vi "Input_channels.vi"(10 "Range":dbl=10.0) -> (0 "error out":errorcluster, 3 "Refnum out":refnum<k21>)   [LabVIEW 2021]
uses:
  <vilib>/DAQmx/create/scale.llb/DAQmx Create Scale (Linear).vi
  <vilib>/DAQmx/create/channels.llb/DAQmx Create Channel (AI-Voltage-Basic).vi
panel:
  out "Numeric":i32
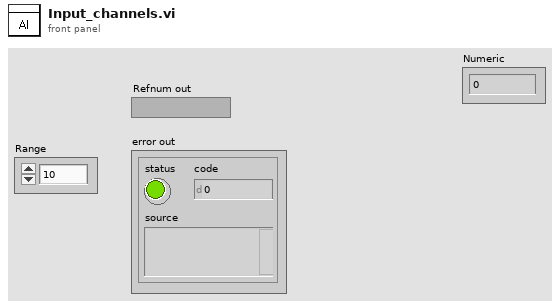
[diagram p1: front panel]
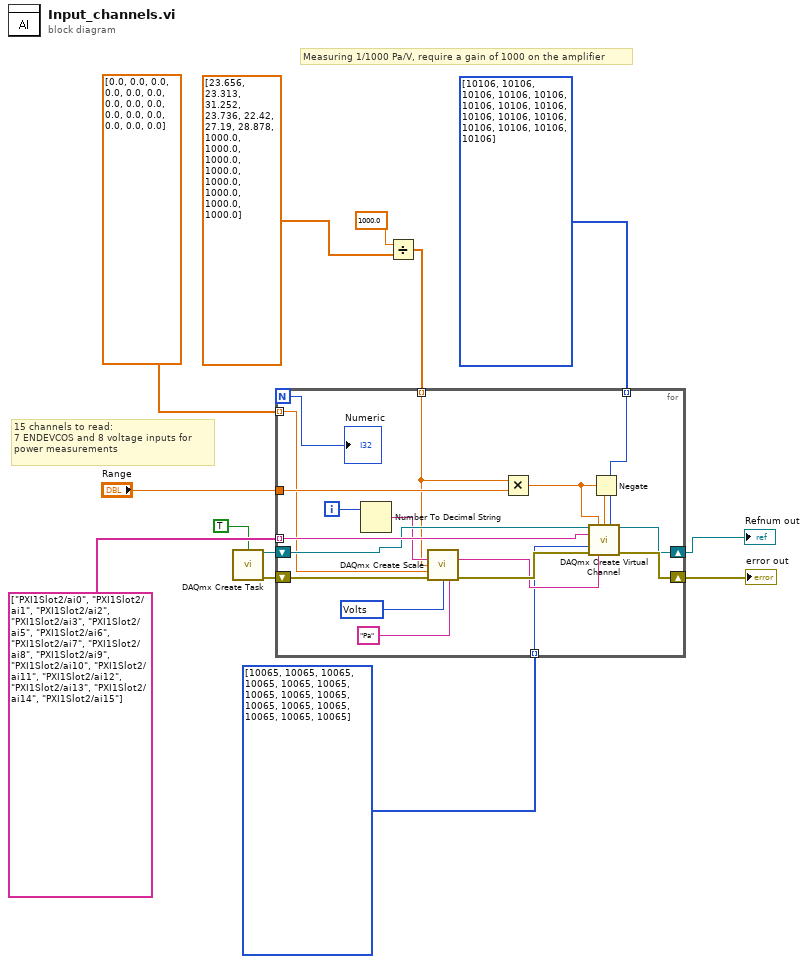
[diagram p0: block diagram]
diagram:
  w5 = i32[] [10065, 10065, 10065, 10065, 10065, 10065, 10065, 10065, 10065, 10065, 10065, 10065, 10065, 10065, 10065] items=["Volts"=10348, "From TEDS"=12516, "From Custom Scale"=10065] ("units")
  w13 = i32[] [10106, 10106, 10106, 10106, 10106, 10106, 10106, 10106, 10106, 10106, 10106, 10106, 10106, 10106, 10106] items=["default"=-1, "RSE"=10083, "NRSE"=10078, "Differential"=10106, "Pseudodifferential"=12529]
  # "15 channels to read:\n7 ENDEVCOS and 8 voltage inputs for \npower measurements"
  # "Measuring 1/1000 Pa/V, require a gain of 1000 on the amplifier"
  n1 = call <vilib>:"DAQmx Create Task.vi"("auto cleanup"=TRUE) -> ("task out"=w9:refnum<k21>, "error out"=w8:errorcluster)  [unwired: 13 in]
  n2 = Divide(x=1000.0, y=dbl[] [23.656, 23.313, 31.252, 23.736, 22.42, 27.19, 28.878, 1000.0, 1000.0, 1000.0, 1000.0, 1000.0, 1000.0, 1000.0, 1000.0]) -> (x/y=w2:dbl[])
  n3 = for {
    N -> [w14]
    tunnel: tag[] ["PXI1Slot2/ai0", "PXI1Slot2/ai1", "PXI1Slot2/ai2", "PXI1Slot2/ai3", "PXI1Slot2/ai5", "PXI1Slot2/ai6", "PXI1Slot2/ai7", "PXI1Slot2/ai8", "PXI1Slot2/ai9", "PXI1Slot2/ai10", "PXI1Slot2/ai11", "PXI1Slot2/ai12", "PXI1Slot2/ai13", "PXI1Slot2/ai14", "PXI1Slot2/ai15"] -> [w30] mode=indexing
    tunnel: w13 -> [w29] mode=indexing
    shift-right: [w31] -> w11
    shift-left: w9 -> [w28]
    shift-right: [w32] -> w10
    shift-left: w8 -> [w26]
    tunnel: "Range" -> [w17]
    tunnel: w5 -> [w23] mode=indexing
    tunnel: w2 -> [w16] mode=indexing
    tunnel: dbl[] [0.0, 0.0, 0.0, 0.0, 0.0, 0.0, 0.0, 0.0, 0.0, 0.0, 0.0, 0.0, 0.0, 0.0, 0.0] -> [w15] mode=indexing
    i -> [w20]
    w22 = 10348 items=["Volts"=10348, "Amps"=10342, "Deg F"=10144, "Deg C"=10143, "Deg R"=10145, "Kelvins"=10325, "Strain"=10299, "Ohms"=10384, "Hz"=10373, "Seconds"=10364, "Meters"=10219, "Inches"=10379, "Degrees"=10146, "Radians"=10273, "g"=10186, "m/s^2"=12470, "Pascals"=10081, "From TEDS"=12516] ("pre-scaled units")
    n4 = Number To Decimal String(number=w20) -> (decimal integer string=w19:string)  [unwired: 1 in]
    n5 = call-poly <vilib>:"DAQmx Create Scale.vi"("name"=w19, "slope"=w16, "y-intercept"=w15, "error in"=w26, "pre-scaled units"=w22, "scaled units"="Pa") -> ("scale out"=w24:tag, "error out"=w25:errorcluster)  [unwired: 8 in]
    n6 = Multiply(x=w16, y=w17) -> (x*y=w18:dbl)
    n7 = Negate(x=w18) -> (-x=w27:dbl)
    n8 = call-poly <vilib>:"DAQmx Create Virtual Channel.vi"("task in"=w28, "maximum value"=w18, "minimum value"=w27, "input terminal configuration"=w29, "physical channels"=w30, "units"=w23, "error in"=w25, "custom scale name"=w24) -> ("task out"=w31:refnum<k21>, "error out"=w32:errorcluster)  [unwired: 6 in]
    "Numeric" <- w14
  }
  "Refnum out" <- w11
  "error out" <- w10
